vi "Hold_subvi.vi"(10 "Pause/Continue":bool, 11 "Boolean in":refnum<vi>) -> ()   [LabVIEW 2020]
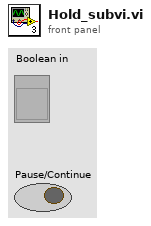
[diagram p1: front panel]
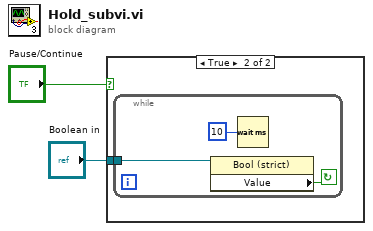
[diagram p0: block diagram]
diagram:
  n1 = case shown="True" "Pause/Continue" {
    tunnel: "Boolean in" -> [_ w3]
    frame False {
    }
    frame True {
      n2 = while {
        tunnel: w3 -> [w4]
        stop <- w6 continue-if-true
        n3 = property class="Bool (strict)"(reference=w4) -> ("Value"=w6:bool)  [unwired: 1 in, 2 out]
        n4 = Wait (ms)(milliseconds to wait=u32 10) -> ()  [unwired: 1 out]
      }
    }
  }
